vi "Display.vi"(8 "error in":errorcluster, 11 "Custom - Timeout in":refnum<class "Custom - Timeout.lvclass">) -> (0 "error out":errorcluster, 3 "Custom - Timeout out":refnum<class "Custom - Timeout.lvclass">)   [LabVIEW 2021, in "Pop-Up.lvlib" / "Custom - Timeout.lvclass"]
doc: "This vi displays the custom timeout Popup.\n\n<b>Code Developed By:</b>\nDaniel Coons\nTechnology Service Corporation\n1983 S Liberty Drive\nBloomington, IN 47403\nPhone: 812 558-7100\ndaniel.coons@tsc.com\nwww.tsc.com/atcs"
uses:
  Custom - Timeout.lvclass
  C:/Development/Open Source/tsc-pop-up/Popup/Popup.lvclass
  <vilib>/Utility/miscctls.llb/LVPositionTypeDef.ctl
  Popup/Popup.lvclass/Popup.ctl
  Custom - Timeout.lvclass/Custom - Timeout.ctl
  Popup/Data Member Access/Read Theme.vi
  Theme/Theme.lvclass
  Popup/Popup.lvclass
  C:/Development/Open Source/tsc-pop-up/PNG/PNG Parent.lvclass
  C:/Development/Open Source/tsc-pop-up/Custom/Custom - Timeout/Custom - Timeout.lvclass
  user32.dll
panel:
  out "header":bool
  out "count":string
  out "2D Picture":picture
  out "Message":string
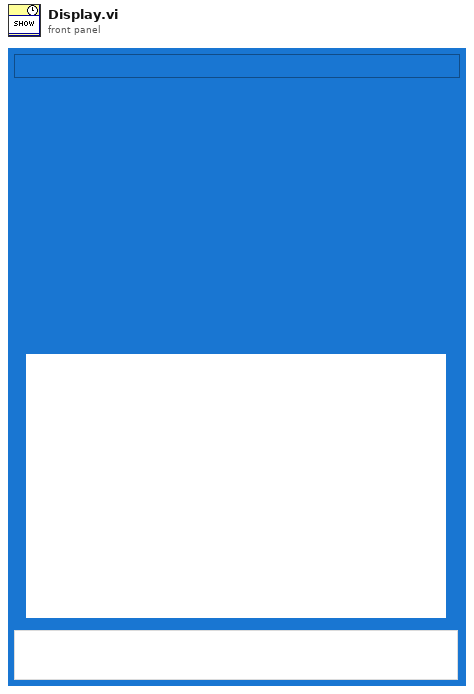
[diagram p1: front panel]
types:
  T1 = typedef "LVPositionTypeDef.ctl" = cluster{"Left":i32, "Top":i32}
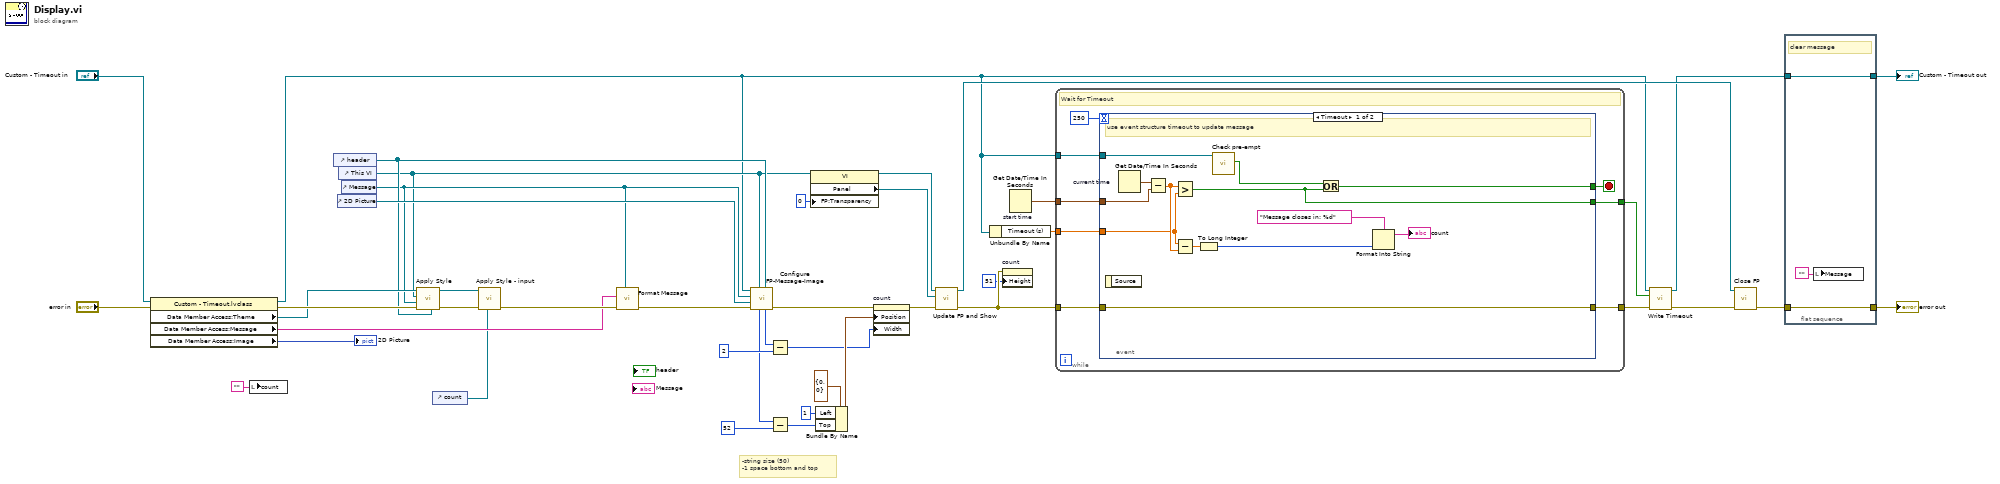
[diagram p0: block diagram]
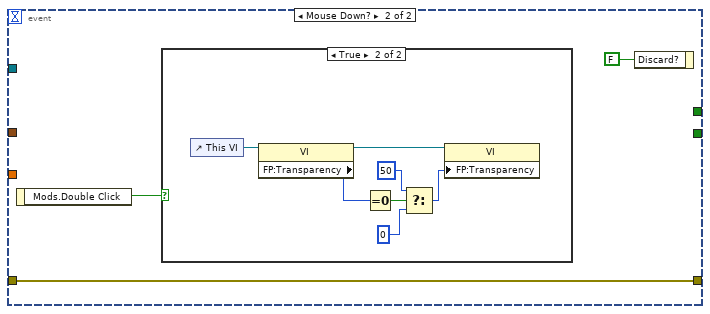
[diagram p2: hidden frame]
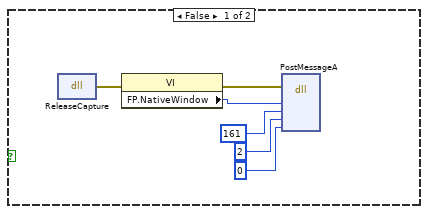
[diagram p3: hidden frame]
diagram:
  # "-string size (50)\n-1 space bottom and top"
  n1 = property class="Custom - Timeout.lvclass"(reference="Custom - Timeout in", error in="error in") -> (reference out=w1:refnum<class "Custom - Timeout.lvclass">, error out=w27:errorcluster, "Data Member Access:Theme"=w26:refnum<class "Theme.lvclass">, "Data Member Access:Message"=w12:string, "Data Member Access:Image"=→"2D Picture":picture)
  n2 = local write "count"("" ("count")) -> ()
  n3 = control-ref of="header"() -> (w16:refnum<vi>)
  n4 = control-ref of="2D Picture"() -> (w23:refnum<vi>)
  n5 = control-ref of="This VI"() -> (w10:refnum<vi>)
  n6 = control-ref of="Message"() -> (w15:refnum<vi>)
  n7 = call "Apply Style.vi"("header ref"=w16, "error in"=w27, "message ref"=w15, "pop up ref"=w10, "Theme in"=w26) -> ("error out"=w17:errorcluster, "Theme out"=w13:refnum<class "Theme.lvclass">)  [unwired: 5 in]
  n8 = control-ref of="count"() -> (w11:refnum<vi>)
  n9 = call "Apply Style - input.vi"("input ref"=w11, "error in (no error)"=w17, "Theme in"=w13) -> ("error out"=w14:errorcluster)  [unwired: 7 in, 1 out]
  n10 = call "Format Message.vi"("formatted string"=w15, "error in"=w14, "String Input"=w12) -> ("error out"=w25:errorcluster)  [unwired: 7 in, 1 out]
  n11 = call "Configure FP-Message-Image.vi"("header ref"=w16, "Pop Up ref"=w10, "error in (no error)"=w25, "Image ref"=w23, "Message ref"=w15, "Popup in"=w1) -> ("error out"=w24:errorcluster, "Panel Width"=w20:i32, "Panel Height"=w18:i32)  [unwired: 1 in, 2 out]
  n12 = Subtract(x=w20, y=2) -> (x-y=w19:i32)
  n13 = Subtract(x=w18, y=52) -> (x-y=w31:i32)
  n14 = property class="VI"(reference=w10, "FP:Transparency"=u8 0 ("Front Panel Window:Transparency")) -> (reference out=w9:refnum<vi>, "Panel"=w8:refnum<vi>)  [unwired: 1 in, 1 out]
  n15 = Bundle By Name(cluster=T1 {"Left"=0, "Top"=0} ("Position"), "Left"=1, "Top"=w31) -> (w30:T1)
  n16 = property on="count" class="Str"(error in=w24, "Position"=w30, "Width"=w19) -> (error out=w22:errorcluster)  [unwired: 1 in, 1 out]
  n17 = call "Update FP and Show.vi"("error in (no error)"=w22, "Panel Ref"=w8, "VI in"=w9) -> ("error out"=w6:errorcluster, "VI out"=w37:refnum<vi>)  [unwired: 7 in]
  n18 = Unbundle By Name(w1) -> ("Timeout (s)"=w41:dbl)
  n19 = property on="count" class="Str"(error in=w6, "Height"=u32 51 ("Size:Height")) -> ()  [unwired: 1 in, 2 out]
  n20 = Get Date/Time In Seconds "start time"() -> (seconds since 1Jan1904=w42:timestamp)
  n21 = while {
    tunnel: [w46] -> w43
    tunnel: w6 -> [w47]
    tunnel: w42 -> [w51]
    tunnel: w41 -> [w49]
    tunnel: w1 -> [w45]
    tunnel: [w44] -> w2
    stop <- w50 stop-if-true
    # "Wait for Timeout"
    n22 = event shown="[0] Timeout" {
      selector: _ -> [_ _]
      dyn-events: _ -> [_ _]
      timeout: 250 -> [_ _]
      tunnel: w51 -> [w64 _]
      tunnel: [w56 _] -> w50
      tunnel: w49 -> [w60 _]
      tunnel: w47 -> [w57 w66]
      tunnel: [w57 w66] -> w46
      tunnel: w45 -> [w54 _]
      tunnel: [w52 _] -> w44
      event Timeout {
        # "use event structure timeout to update message"
        n23 = event-data() -> ()  [unwired: 1 in, 1 out]
        n24 = Get Date/Time In Seconds "current time"() -> (seconds since 1Jan1904=w63:timestamp)
        n25 = Subtract(x=w63, y=w64) -> (x-y=w62:dbl)
        n26 = Greater?(x=w62, y=w60) -> (0:w52:bool)
        n27 = Subtract(x=w60, y=w62) -> (x-y=w61:dbl)
        n28 = To Long Integer(number=w61) -> (32bit integer=w58:i32)
        n29 = call "Check pre-empt.vi"("_Popup in"=w54) -> ("Pre-empted?"=w55:bool)  [unwired: 8 in, 2 out]
        n30 = Or(x=w55, y=w52) -> (x .or. y?=w56:bool)
        n31 = Format Into String(format string="Message closes in: %d", w58) -> (resulting string=→"count":string)  [unwired: 2 in, 1 out]
      }
      event Mouse Down? {
        n32 = event-data() -> ("Mods.Double Click"=w65:bool)  [unwired: 1 in]
        n33 = case shown="True" w65 {
          frame False {
            n34 = dll-call lib="user32.dll" fn="ReleaseCapture"() -> (error out=w71:errorcluster)  [unwired: 4 in, 1 out]
            n35 = property class="VI"(error in=w71) -> (error out=w72:errorcluster, "FP.NativeWindow"=w73:u64)  [unwired: 1 in, 1 out]
            n36 = dll-call lib="user32.dll" fn="PostMessageA"(error in=w72, "hWnd"=w73, "Msg"=161, "wParam"=2, "lParam"=0) -> ()  [unwired: 7 in, 2 out]
          }
          frame True {
            n37 = control-ref of="This VI"() -> (w80:refnum<vi>)
            n38 = property class="VI"(reference=w80) -> (reference out=w78:refnum<vi>, "FP:Transparency"=w79:u8)  [unwired: 1 in, 1 out]
            n39 = Equal To 0?(x=w79) -> (x = 0?=w77:bool)
            n40 = Select(t=u8 50, s=w77, f=u8 0) -> (s? t:f=w76:u8)
            n41 = property class="VI"(reference=w78, "FP:Transparency"=w76) -> ()  [unwired: 1 in, 2 out]
          }
        }
        n42 = event-data("Discard?"=FALSE) -> ()  [unwired: 1 in, 1 out]
      }
    }
  }
  n43 = call "Write Timeout.vi"("error in (no error)"=w43, "Timeout?"=w2, "Popup in"=w1) -> ("error out"=w4:errorcluster, "Popup out"=w3:refnum<class "Custom - Timeout.lvclass">)  [unwired: 7 in]
  n44 = call "Close FP.vi"("error in (no error)"=w4, "VI in"=w37) -> ("error out"=w36:errorcluster)  [unwired: 9 in]
  n45 = flat-sequence {
    tunnel: w36 -> [w83]
    tunnel: [w83] -> w35
    tunnel: w3 -> [w82]
    tunnel: [w82] -> w34
    frame #0 {
      # "clear message"
      n46 = local write "Message"("" ("Message")) -> ()
    }
  }
  "error out" <- w35
  "Custom - Timeout out" <- w34
